vi "Log_beam_power.vi"(3 "Message":string, 4 "Beam Names":string[](array[string]), 5 "Beam Data":dbl[][](array[numeric]) format="%.2f") -> (2 "Power History":dbl[][](array[numeric]))   [LabVIEW 2020]
uses:
  ADAM Client/Sub VIs/ADAM Controls/Channel_names.ctl
panel:
  out "Log File":path
  # "X                Y                 Z                 Power"
  # "Green Unshifted\nGreen Shifted\nBlue Unshifted\nBlue Shifted"
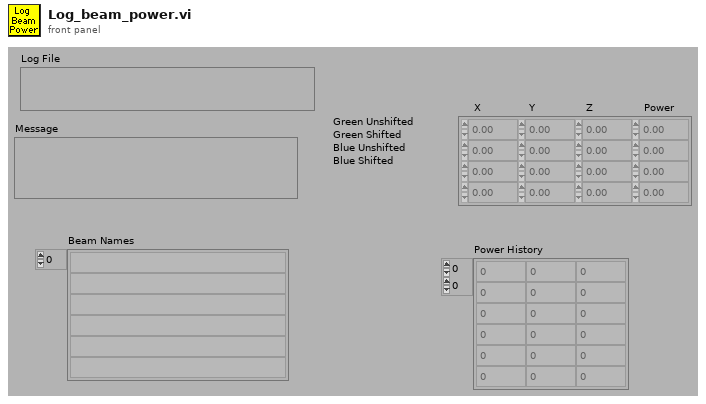
[diagram p1: front panel]
types:
  T1 = typedef "Channel_names.ctl" = enum16{"Active Only", "Active + Off", "All Channels"}
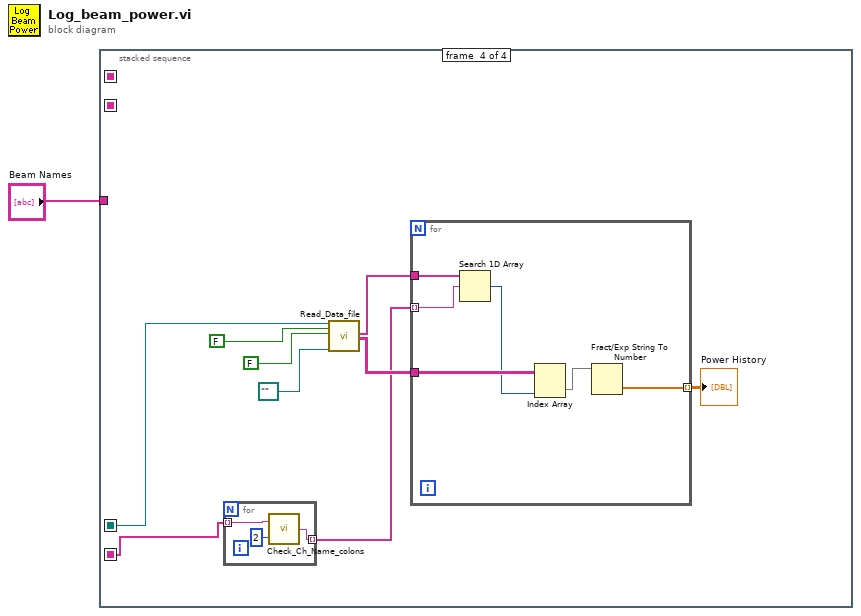
[diagram p0: block diagram]
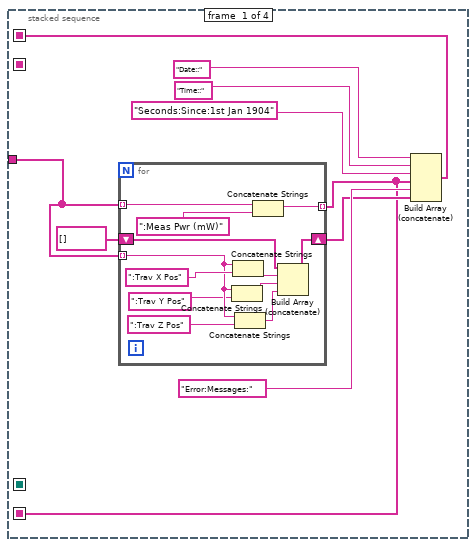
[diagram p2: hidden frame]
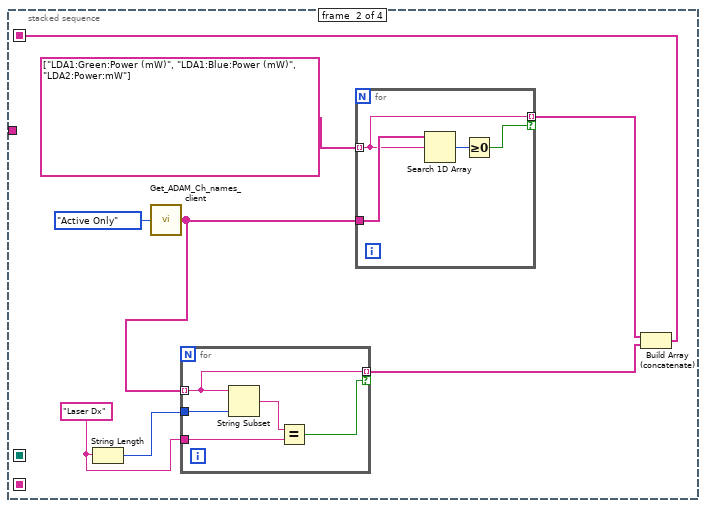
[diagram p3: hidden frame]
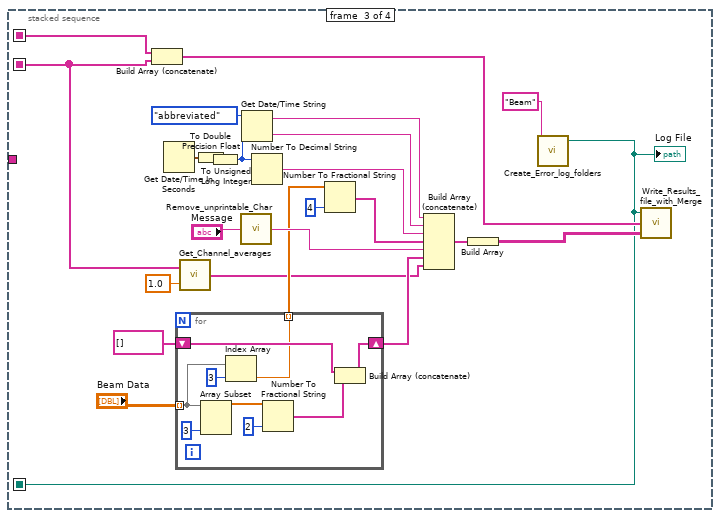
[diagram p4: hidden frame]
diagram:
  n1 = stacked-sequence {
    seq-local: [_ w23 _ _] -> [_ _ w43 _]
    seq-local: [w3 _ _ _] -> [_ _ w44 _]
    seq-local: [w2 _ _ _] -> [_ _ _ w74]
    seq-local: [_ _ w40 _] -> [_ _ _ w81]
    tunnel: "Beam Names" -> [w4 _ _ _]
    frame #0 {
      n2 = for {
        tunnel: w4 -> [w22] mode=indexing
        tunnel: [w20] -> w2 mode=indexing
        shift-right: [w11] -> w5
        shift-left: string[] [] -> [w15]
        tunnel: w4 -> [w18] mode=indexing
        n3 = Concatenate Strings(w18, ":Trav Y Pos") -> (w13:string)
        n4 = Concatenate Strings(w18, ":Trav X Pos") -> (w14:string)
        n5 = Concatenate Strings(w18, ":Trav Z Pos") -> (w12:string)
        n6 = Concatenate Strings(w22, ":Meas Pwr (mW)") -> (w20:string)
        n7 = Build Array (concatenate)(w15, w14, w13, w12) -> (w11:string[])
      }
      n8 = Build Array (concatenate)("Date::", "Time::", "Seconds:Since:1st Jan 1904", w2, "Error:Messages:", w5) -> (w3:string[])
    }
    frame #1 {
      w27 = "Laser Dx"
      n9 = String Length(string=w27) -> (length=w28:i32)
      n10 = call "Get_ADAM_Ch_names_client.vi"("Channel names set"=Channel_names."Active Only") -> ("Ch names"=w29:string[])
      n11 = for {
        tunnel: w29 -> [w32] mode=indexing
        tunnel: w28 -> [w35]
        tunnel: w27 -> [w33]
        tunnel: [w32] -> w24 mode=indexing if=w31
        n12 = String Subset(string=w32, length (rest)=w35) -> (substring=w34:string)  [unwired: 1 in]
        n13 = Equal?(x=w34, y=w33) -> (x = y?=w31:bool)
      }
      n14 = for {
        tunnel: w29 -> [w39]
        tunnel: string[] ["LDA1:Green:Power (mW)", "LDA1:Blue:Power (mW)", "LDA2:Power:mW"] -> [w37] mode=indexing
        tunnel: [w37] -> w25 mode=indexing if=w36
        n15 = Search 1D Array(1D array=w39, element=w37) -> (index of element=w38:i32)  [unwired: 1 in]
        n16 = Greater Or Equal To 0?(x=w38) -> (x >= 0?=w36:bool)
      }
      n17 = Build Array (concatenate)(w25, w24) -> (w23:string[])
    }
    frame #2 {
      n18 = Build Array (concatenate)(w44, w43) -> (w42:string[])
      n19 = Get Date/Time In Seconds() -> (seconds since 1Jan1904=w48:timestamp)
      n20 = for {
        shift-right: [w71] -> w50
        shift-left: string[] [] -> [w72]
        tunnel: "Beam Data" -> [w65] mode=indexing
        tunnel: [w64] -> w51 mode=indexing
        n21 = Array Subset(array=w65, length=3 ("Array Length")) -> (w68:dbl[])  [unwired: 1 in]
        n22 = Index Array(array=w65, index=3 ("Index")) -> (element=w64:dbl)
        n23 = Number To Fractional String(number=w68, precision (6)=i16 2) -> (F-format string=w69:string[])  [unwired: 2 out]
        n24 = Build Array (concatenate)(w72, w69) -> (w71:string[])
      }
      n25 = call "Get_Channel_averages.vi"("Desired Ch Names"=w43, "Averaging time (mins)"=1.0) -> ("Values"=w47:string[])  [unwired: 1 in, 2 out]
      n26 = To Double Precision Float(number=w48) -> (double precision float=w61:dbl)
      n27 = To Unsigned Long Integer(number=w61) -> (unsigned 32bit integer=w60:u32)
      n28 = call "Remove_unprintable_Char.vi"("Input String"="Message") -> ("Output String"=w54:string)
      n29 = Get Date/Time String(date format (0)=enum16{"short", "long", "abbreviated"}."abbreviated", seconds (now)=w60) -> (date string=w59:string, time string=w58:string)  [unwired: 1 out]
      n30 = Number To Decimal String(number=w60) -> (decimal integer string=w57:string)  [unwired: 1 out]
      n31 = Number To Fractional String(number=w51, precision (6)=i16 4) -> (F-format string=w55:string[])  [unwired: 2 out]
      n32 = Build Array (concatenate)(w59, w58, w57, w55, w54, w50, w47) -> (w46:string[])
      n33 = Build Array(w46) -> (w45:string[][])
      n34 = call "Create_Error_log_folders.vi"("Log Filename"="Beam" ("Input Element")) -> ("Local Log File"=w40:path)  [unwired: 5 in, 1 out]
      "Log File" <- w40
      n35 = call "Write_Results_file_with_Merge.vi"("Values In"=w45, "Channel Names in"=w42, "Filename"=w40) -> ()  [unwired: 1 in, 2 out]
    }
    frame #3 {
      n36 = for {
        tunnel: w74 -> [w84] mode=indexing
        tunnel: [w82] -> w73 mode=indexing
        n37 = call "Check_Ch_Name_colons.vi"("No of Colons"=2, "Ch Name in"=w84) -> ("Ch Name out"=w82:string)
      }
      n38 = call "Read_Data_file.vi"("Results file"=w81, "Read Channel Names only"=FALSE, "Delete First Rows?"=FALSE, "Template File"=path "") -> ("Ch names Out"=w77:string[], "Channel Values Out"=w76:string[][])  [unwired: 5 in, 9 out]
      n39 = for {
        tunnel: w73 -> [w90] mode=indexing
        tunnel: w77 -> [w89]
        tunnel: w76 -> [w88]
        tunnel: [w85] -> w75 mode=indexing
        n40 = Search 1D Array(1D array=w89, element=w90) -> (index of element=w87:i32)  [unwired: 1 in]
        n41 = Index Array(array=w88, index (col)=w87) -> (element=w86:string[])  [unwired: 1 in]
        n42 = Fract/Exp String To Number(string=w86) -> (number=w85:dbl[])  [unwired: 3 in, 1 out]
      }
      "Power History" <- w75
    }
  }
